vi "Set Pre Amplification.vi"(8 "error in (no error)":errorcluster, 11 "CCDCamera in":refnum<class "Real Camera.lvclass">) -> (0 "error out":errorcluster, 3 "CCDCamera out":refnum<class "Real Camera.lvclass">)   [LabVIEW 2018, in "Real Camera.lvclass"]
doc: "Set pre amplification (1x or 2x)"
uses:
  Real Camera.lvclass
  C:/Users/Denis/Desktop/S4ACS/S4ACS/Simulated_CCD_Camera/Simulated Camera.lvclass
  Simulated_CCD_Camera/Simulated Camera.lvclass
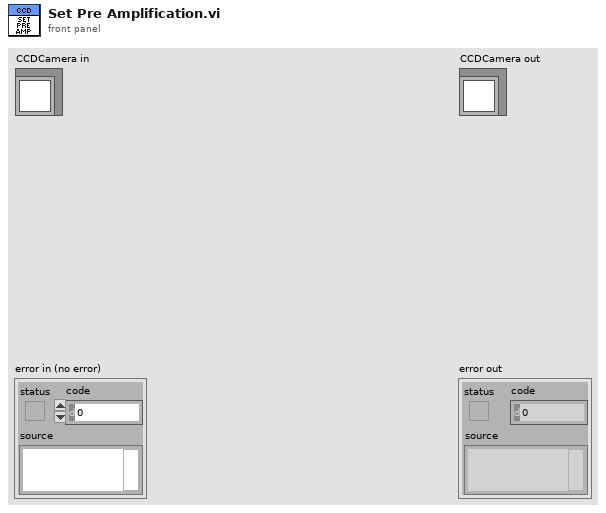
[diagram p1: front panel]
types:
  T1 = cluster{"PREAMP":u16, "READOUT_RATE":u16, "EM_GAIN":u16, "VERTICAL_SHIFT_SPEED":u16, "READ_MODE":u16, "FRAME_TRANSFER":bool, "VERTICAL_CLOCK_VOLTAGE":u16, "ACQUISITION_MODE":u16, "AD_CHANNEL":u16, "EM_MODE":u16, "SHUTTER_TTL":u16, "SHUTTER_OPENING_TIME":u16, "SHUTTER_CLOSING_TIME":u16, "SHUTTER_MODE":u16, "TRIGGER_MODE":u16, "VBIN":u16, "INITIAL_LINE":u16, "INITIAL_COLUMN":u16, "FINAL_LINE":u16, "FINAL_COLUMN":u16, "HBIN":u16}
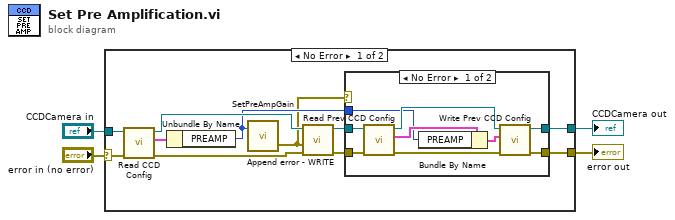
[diagram p0: block diagram]
diagram:
  n1 = case shown="No Error" "error in (no error)" {
    selector: "error in (no error)" -> [w15 w28]
    tunnel: [w7 w28] -> w4
    tunnel: [w8 w27] -> w3
    tunnel: "CCDCamera in" -> [w13 w27]
    frame No Error {
      n2 = call "Read CCD Config.vi"("error in (no error)"=w15, "CCDCamera in"=w13) -> ("error out"=w12:errorcluster, "CCD Config"=w14:T1, "CCDCamera out"=w11:refnum<class "Real Camera.lvclass">)  [unwired: 7 in]
      n3 = Unbundle By Name(w14) -> ("PREAMP"=w6:u16)
      n4 = call <userlib>:"SetPreAmpGain.vi"("index"=w6) -> ("error out"=w5:errorcluster)  [unwired: 1 in, 1 out]
      n5 = call "Append error - WRITE.vi"("error in (no error)"=w12, "error"=w5, "Simulated_CCD_Camera in"=w11) -> ("error out"=w10:errorcluster, "Simulated_CCD_Camera out"=w9:refnum<class "Real Camera.lvclass">)  [unwired: 7 in]
      n6 = case shown="No Error" w5 {
        tunnel: [w23 w26] -> w8
        tunnel: [w21 w25] -> w7
        tunnel: w10 -> [w18 w25]
        tunnel: w9 -> [w17 w26]
        tunnel: w6 -> [w16 _]
        frame No Error {
          n7 = call-dynamic "Read Prev CCD Config.vi"("error in (no error)"=w18, "Simulated_CCD_Camera in"=w17) -> ("error out"=w22:errorcluster, "Prev CCD Config"=w20:T1, "Simulated_CCD_Camera out"=w24:refnum<class "Real Camera.lvclass">)  [unwired: 7 in]
          n8 = Bundle By Name(cluster=w20, "PREAMP"=w16) -> (w19:T1)
          n9 = call-dynamic "Write Prev CCD Config.vi"("error in (no error)"=w22, "Prev CCD Config"=w19, "Simulated_CCD_Camera in"=w24) -> ("error out"=w21:errorcluster, "Simulated_CCD_Camera out"=w23:refnum<class "Real Camera.lvclass">)  [unwired: 7 in]
        }
        frame Error {
        }
      }
    }
    frame Error {
    }
  }
  "error out" <- w4
  "CCDCamera out" <- w3
